vi "Example.vi"() -> ()   [LabVIEW 2020]
uses:
  <userlib>/lvwamp/WAMP Client/WAMP Client.lvclass
panel:
  in  "Realm":string="test"
  in  "Publish Array Payload":i32[](array[numeric])
  in  "Topic URI":string="test.topic"
  in  "Publish":bool caption="Publish Topic"
  in  "Port":u16=8080
  in  "Router Address":string="localhost"
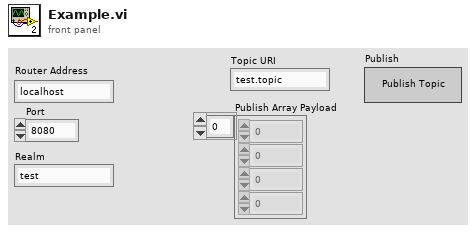
[diagram p1: front panel]
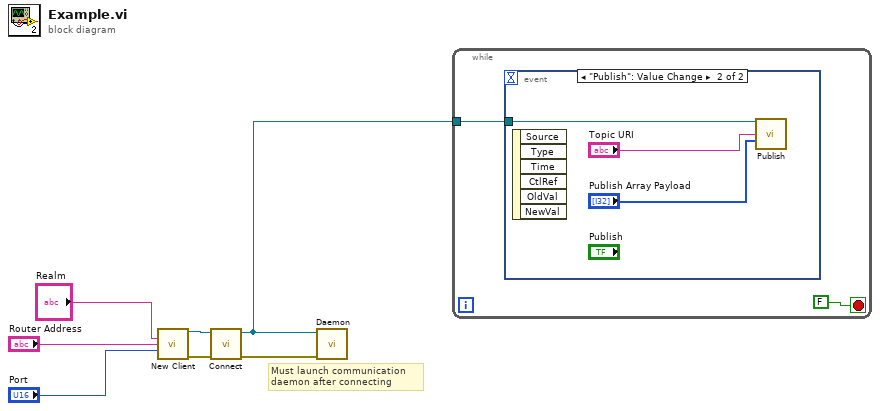
[diagram p0: block diagram]
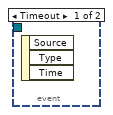
[diagram p2: hidden frame]
diagram:
  # "Must launch communication \ndaemon after connecting"
  n1 = call <userlib>:"New Client.vi"("Realm"="Realm", "Address"="Router Address", "Port"="Port") -> ("reference out"=w5:refnum<class "WAMP Client.lvclass">, "error out"=w4:errorcluster)  [unwired: 11 in]
  n2 = call <userlib>:"Connect.vi"("error in (no error)"=w4, "WAMP Client in"=w5) -> ("error out"=w2:errorcluster, "WAMP Client out"=w1:refnum<class "WAMP Client.lvclass">)  [unwired: 8 in]
  n3 = call-dynamic "Daemon.vi"("error in (no error)"=w2, "WAMP Client in"=w1) -> ()  [unwired: 8 in, 2 out]
  n4 = while {
    tunnel: w1 -> [w9]
    stop <- FALSE stop-if-true
    n5 = event shown="[1] \"Publish\": Value Change" {
      selector: _ -> [_ _]
      dyn-events: _ -> [_ _]
      timeout: _ -> [_ _]
      tunnel: w9 -> [_ w12]
      event Timeout {
        n6 = event-data() -> ()  [unwired: 1 in, 3 out]
      }
      event "Publish": Value Change {
        n7 = event-data() -> ()  [unwired: 1 in, 6 out]
        n8 = call-dynamic "Publish.vi"("WAMP Client in"=w12, "Topic URI"="Topic URI", "Arguments"="Publish Array Payload") -> ()  [unwired: 11 in, 2 out]
      }
    }
  }
